vi "Drag.vi"(0 "FSM.Label In":refnum<class "FSM.Label.lvclass">, 9 "delta":T1) -> (4 "FSM.Label Out":refnum<class "FSM.Label.lvclass">)   [LabVIEW 2020, in "FSM.Label.lvclass"]
uses:
  FSM.Label.lvclass
  <vilib>/Utility/miscctls.llb/LVPoint32TypeDef.ctl
  FSM.Label.lvclass/FSM.Label.ctl
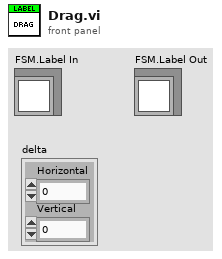
[diagram p1: front panel]
types:
  T1 = typedef "LVPoint32TypeDef.ctl" = cluster{"Horizontal":i32, "Vertical":i32}
  T2 = cluster{"left":i16, "top":i16, "right":i16, "bottom":i16}
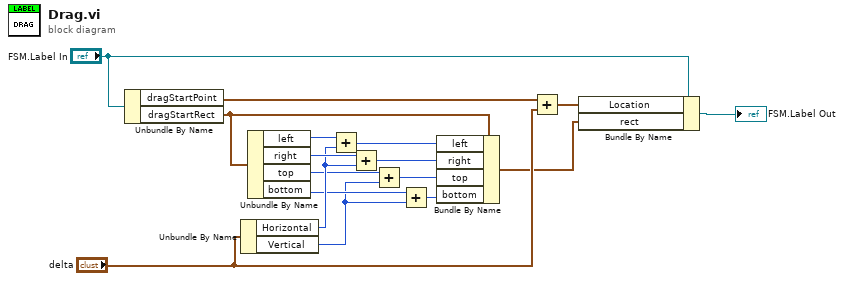
[diagram p0: block diagram]
diagram:
  n1 = Unbundle By Name("FSM.Label In") -> ("dragStartPoint"=w17:cluster{"x":i16, "y":i16}, "dragStartRect"=w10:T2)
  n2 = Unbundle By Name("delta") -> ("Horizontal"=w11:i32, "Vertical"=w1:i32)
  n3 = Unbundle By Name(w10) -> ("left"=w14:i16, "right"=w13:i16, "top"=w5:i16, "bottom"=w3:i16)
  n4 = Add(x=w14, y=w11) -> (x+y=w9:i32)
  n5 = Add(x=w13, y=w11) -> (x+y=w8:i32)
  n6 = Add(x=w5, y=w1) -> (x+y=w4:i32)
  n7 = Add(x=w3, y=w1) -> (x+y=w2:i32)
  n8 = Bundle By Name(cluster=w10, "left"=w9, "right"=w8, "top"=w4, "bottom"=w2) -> (w7:T2)
  n9 = Add(x=w17, y="delta") -> (x+y=w15:T1)
  n10 = Bundle By Name(cluster="FSM.Label In", "Location"=w15, "rect"=w7) -> (→"FSM.Label Out":refnum<class "FSM.Label.lvclass">)
